vi "3D Graph-Ran.vi"() -> ()   [LabVIEW 2012]
uses:
  <vilib>/Native 3D Graph/xcontrol/3DPC_SurfacePlot.xctl
  <vilib>/Math Plots/3D Math Plots/3D Scatter/3D Scatter XCtrl/3D Scatter.xctl
  <vilib>/Math Plots/3D Math Plots/3D Stem/3D Stem XCtrl/3D Stem.xctl
  <vilib>/Math Plots/3D Math Plots/3D Stem/3D Stem Datatype/Public/Plot Helper (Vector).vi
  <vilib>/Math Plots/3D Math Plots/3D Scatter/3D Scatter Datatype/Public/Plot Helper (Vector).vi
  <vilib>/Math Plots/3D Math Plots/3D Scatter/3D Scatter Datatype/3D Scatter Datatype.lvclass
  <vilib>/Math Plots/3D Math Plots/3D Stem/3D Stem Datatype/3D Stem Datatype.lvclass
panel:
  out "Numeric":i32
  out "array of numbers or points":dbl[](array[numeric])
  in  "Interpolate":i32
  out "y value 2":dbl
  out "3D Picture":refnum<vi>(3d-picture)
  out "3D Stem":refnum<class "3D Plot Datatype.lvclass">[](xcontrol)
  out "3D Scatter":refnum<class "3D Plot Datatype.lvclass">[](xcontrol)
  out "3D Graph":refnum<class "Base Datatype.lvclass">[](xcontrol)
  in  "z value":dbl
  in  "y value":dbl
  in  "x value":dbl
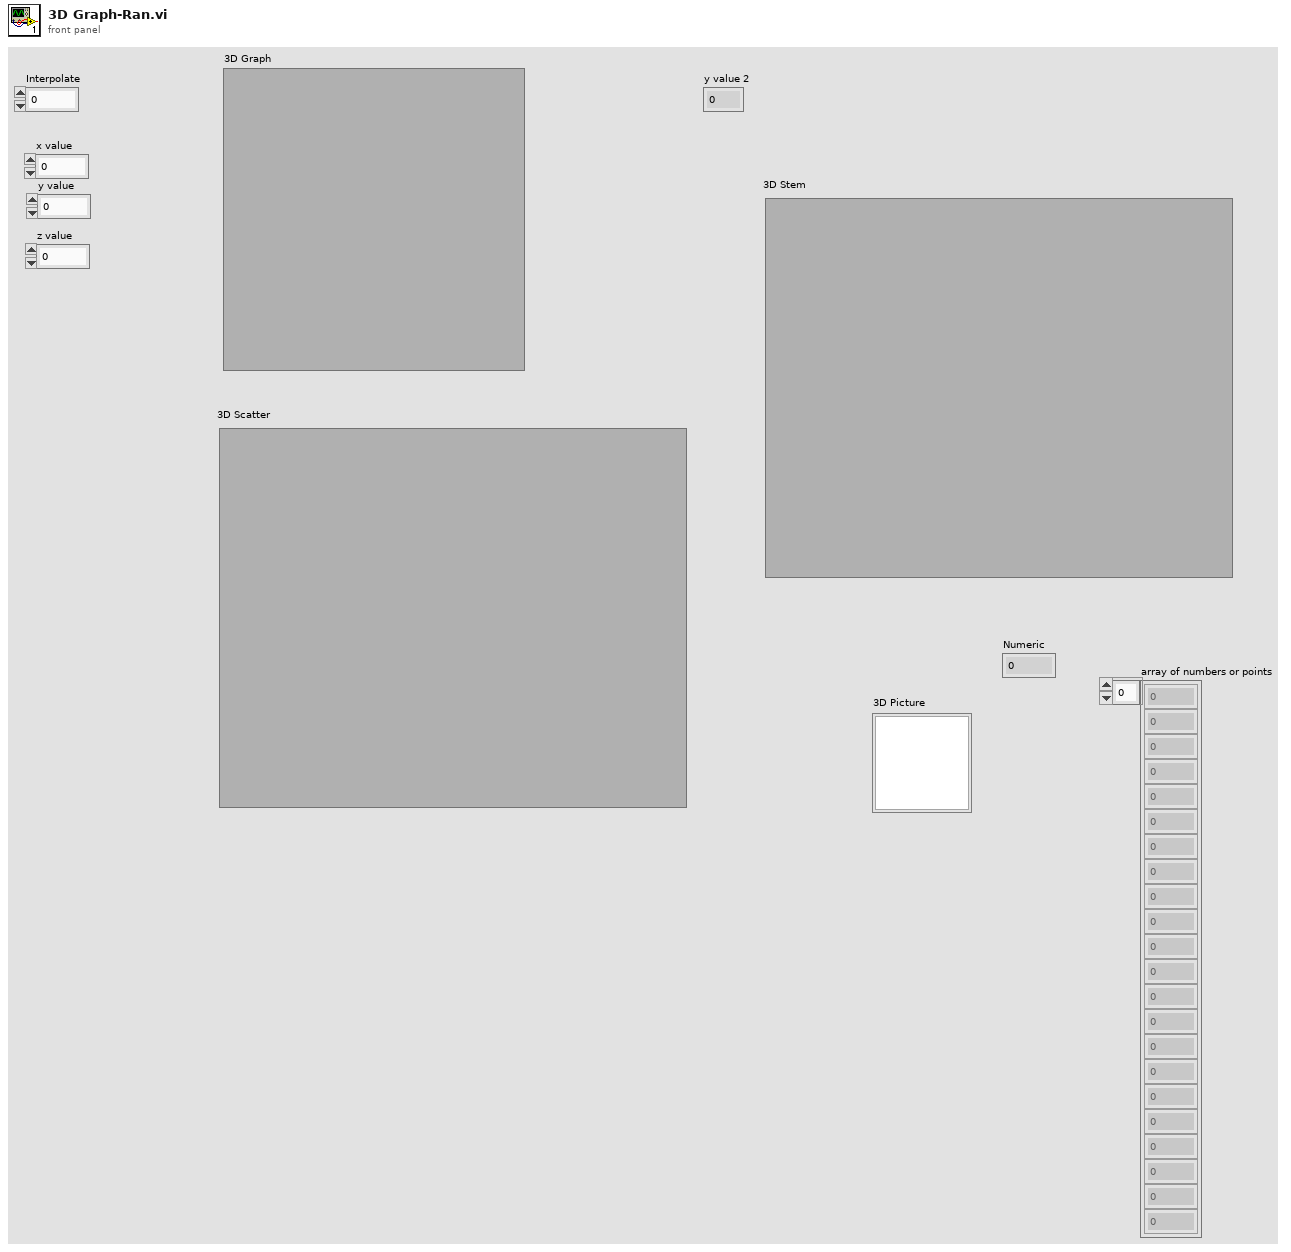
[diagram p1: front panel]
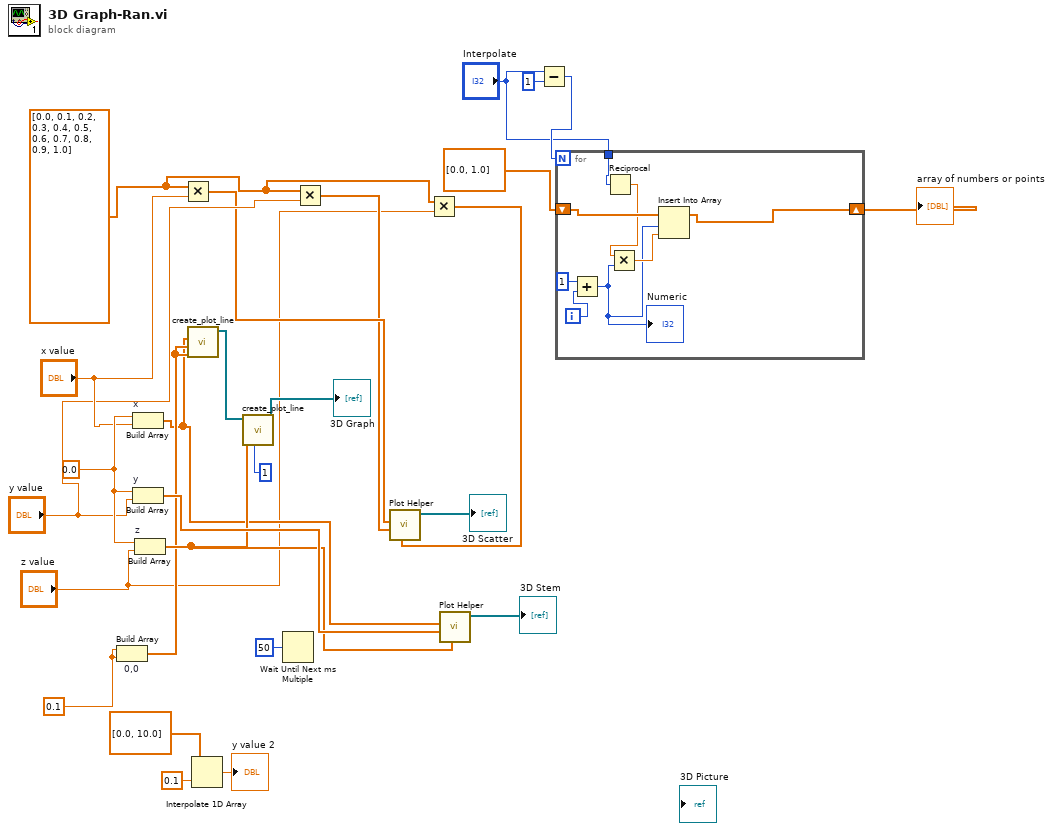
[diagram p0: block diagram]
diagram:
  w8 = dbl[] [0.0, 0.1, 0.2, 0.3, 0.4, 0.5, 0.6, 0.7, 0.8, 0.9, 1.0] ("array of numbers or points")
  w17 = 0.1 ("element")
  w20 = 0.0 ("element")
  n1 = Build Array "0,0"(w17, w17) -> (w19:dbl[])
  n2 = Build Array "x"(w20, "x value") -> (w13:dbl[])
  n3 = Build Array "y"(w20, "y value") -> (w22:dbl[])
  n4 = Build Array "z"(w20, "z value") -> (w21:dbl[])
  n5 = Multiply(x=w8, y="x value") -> (x*y=w10:dbl[])
  n6 = call <vilib>:"create_plot_line.vi"("z vector"=w19, "y vector"=w19, "x vector"=w13) -> ("plots out"=w18:refnum<class "Base Datatype.lvclass">[])  [unwired: 2 in, 6 out]
  n7 = Interpolate 1D Array(1:0.1 ("fractional index or x"), 2:dbl[] [0.0, 10.0] ("array of numbers or points")) -> (0:→"y value 2":dbl)
  n8 = call <vilib>:"create_plot_line.vi"("plot ID"=1, "z vector"=w21, "plots in"=w18) -> ("plots out"=→"3D Graph":refnum<class "Base Datatype.lvclass">[])  [unwired: 2 in, 6 out]
  n9 = Wait Until Next ms Multiple(millisecond multiple=u32 50) -> ()  [unwired: 1 out]
  n10 = Multiply(x=w8, y="y value") -> (x*y=w9:dbl[])
  n11 = Multiply(x=w8, y="z value") -> (x*y=w6:dbl[])
  n12 = call-poly <vilib>:"Plot Helper.vi"("z vector"=w6, "y vector"=w9, "x vector"=w10) -> ("3D Plot lvclass Array out"=→"3D Scatter":refnum<class "3D Plot Datatype.lvclass">[])  [unwired: 3 in, 5 out]
  n13 = call-poly <vilib>:"Plot Helper.vi"("z vector"=w21, "y vector"=w22, "x vector"=w13) -> ("3D Plot lvclass Array out"=→"3D Stem":refnum<class "3D Plot Datatype.lvclass">[])  [unwired: 3 in, 5 out]
  n14 = Subtract(x="Interpolate", y=1) -> (x-y=w3:i32)
  n15 = for {
    N: w3 -> [_]
    shift-right: [w32] -> w4
    shift-left: dbl[] [0.0, 1.0] ("array of numbers or points") -> [w35]
    tunnel: "Interpolate" -> [w31]
    i -> [w30]
    n16 = Add(x=1, y=w30) -> (x+y=w28:i32)
    "Numeric" <- w28
    n17 = Reciprocal(x=w31) -> (1/x=w34:dbl)
    n18 = Multiply(x=w34, y=w28) -> (x*y=w33:dbl)
    n19 = Insert Into Array(array=w35, index=w28, new element=w33) -> (w32:dbl[])
  }
  "array of numbers or points" <- w4
